vi "Device Settings Window.vi"(8 "Error In":errorcluster) -> (0 "Error Out":errorcluster)   [LabVIEW 2019]
uses:
  Controls/Device Settings.ctl
panel:
  in  "Device Settings":T1={"Device Type"="", "Device Name"="", "DAQmx Name"="Dev1", "Terminal Wiring"=10106} {"Terminal Wiring" items=["Default"=-1, "RSE"=10083, "NRSE"=10078, "Differential"=10106, "Pseudodifferential"=12529]}
  in  "Cancel Button":bool
  in  "OK Button":bool
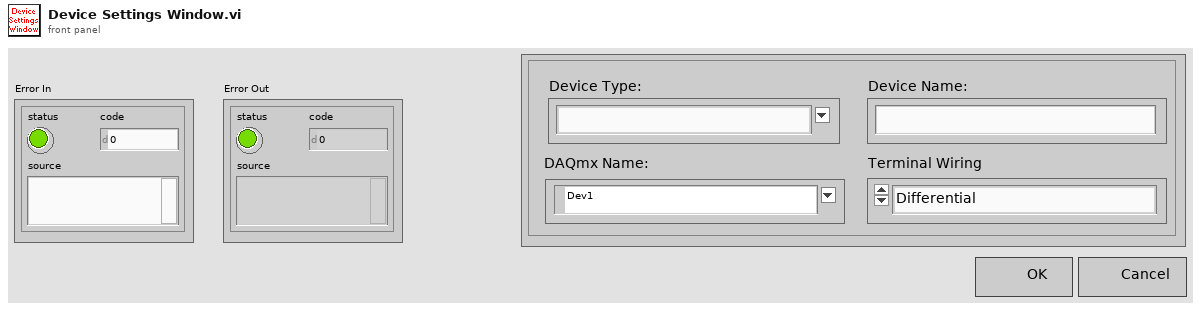
[diagram p1: front panel]
types:
  T1 = typedef "Device Settings.ctl" = cluster{"Device Type":string, "Device Name":string, "DAQmx Name":tag, "Terminal Wiring":i32}
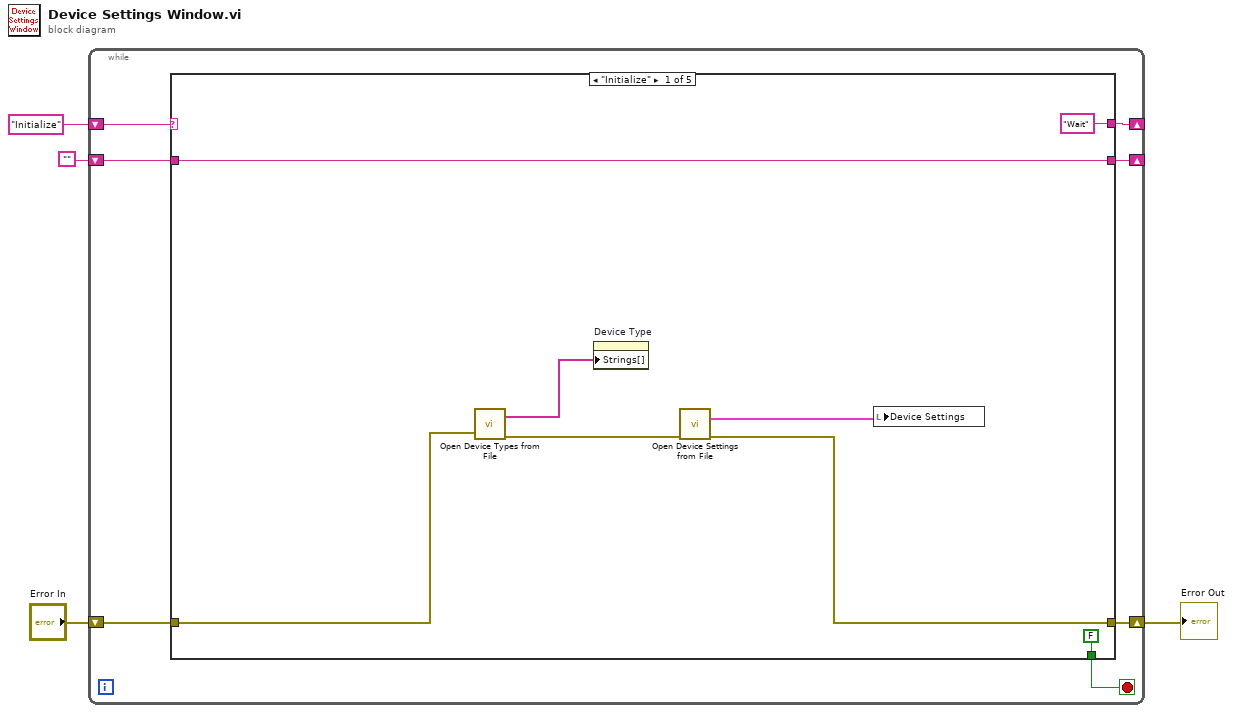
[diagram p0: block diagram]
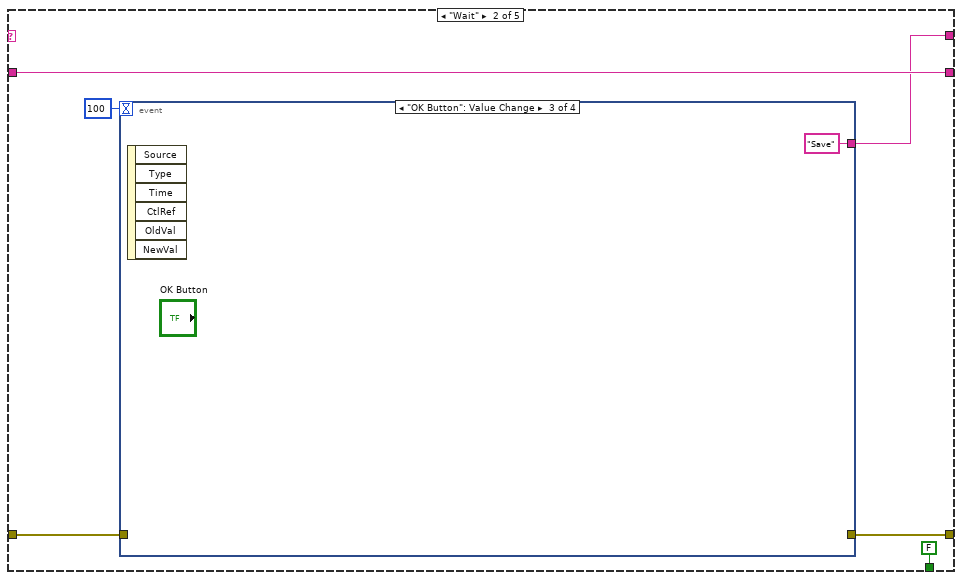
[diagram p2: hidden frame]
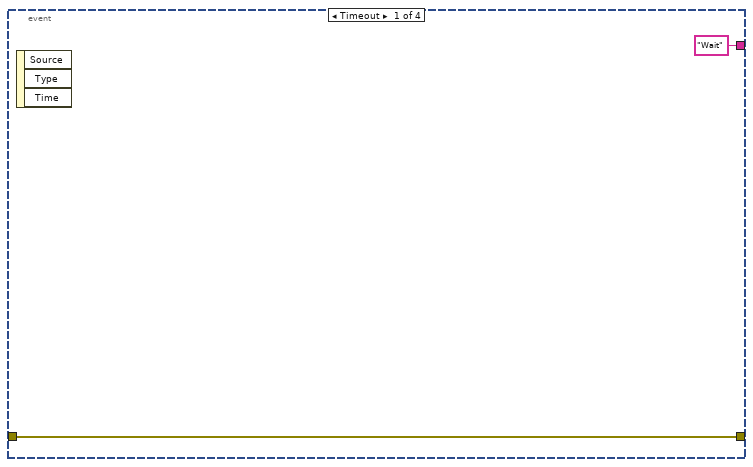
[diagram p3: hidden frame]
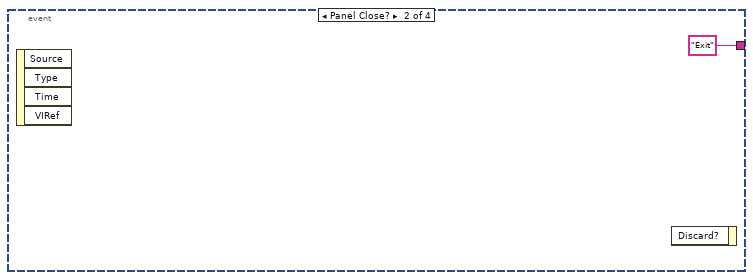
[diagram p4: hidden frame]
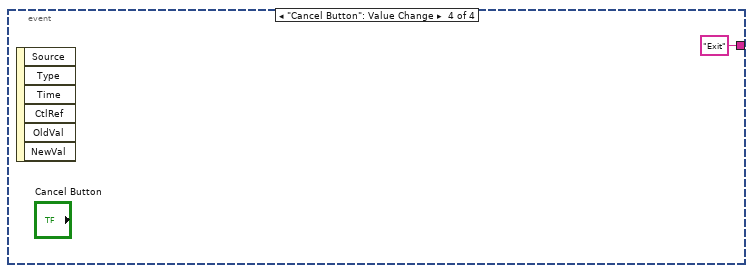
[diagram p5: hidden frame]
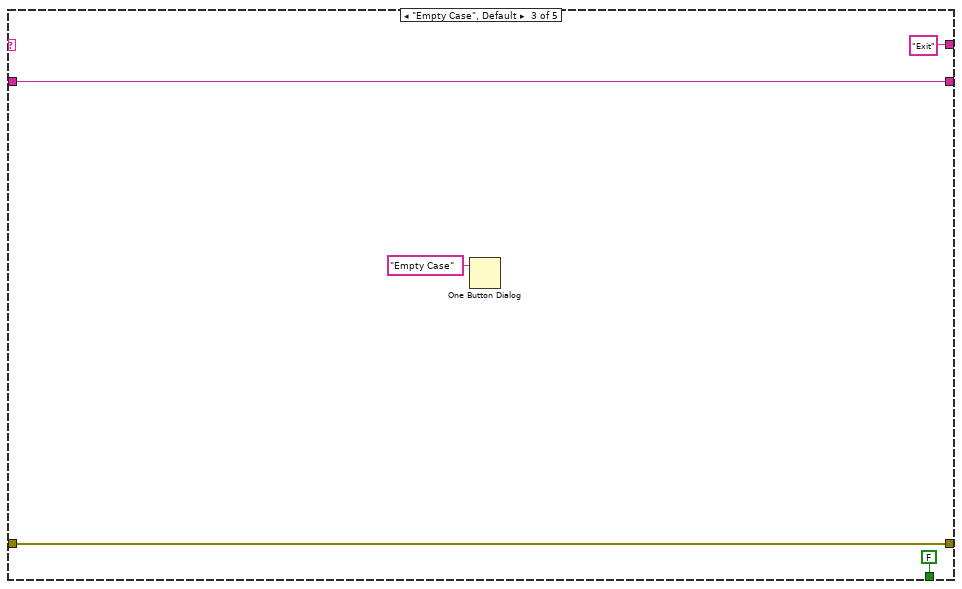
[diagram p6: hidden frame]
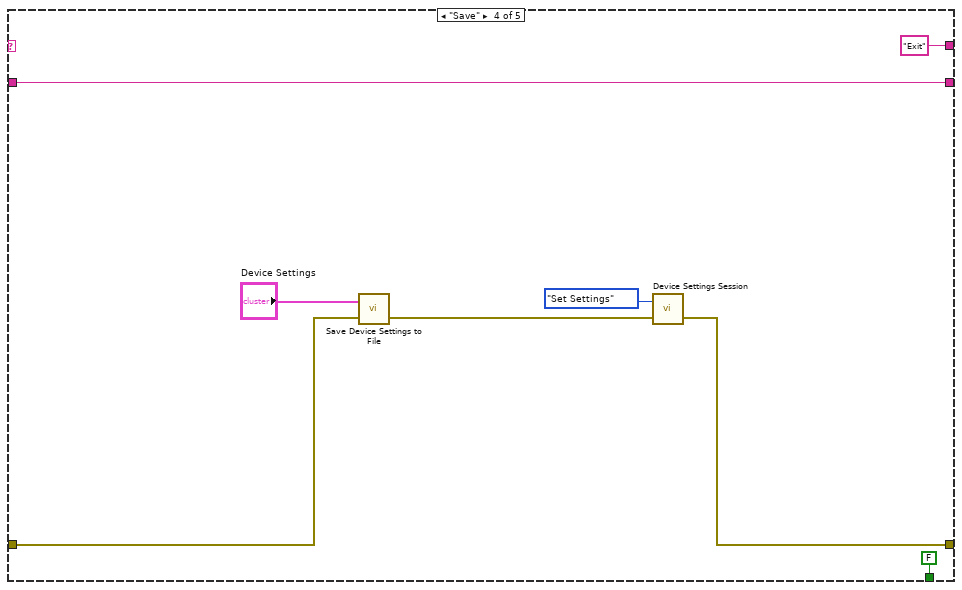
[diagram p7: hidden frame]
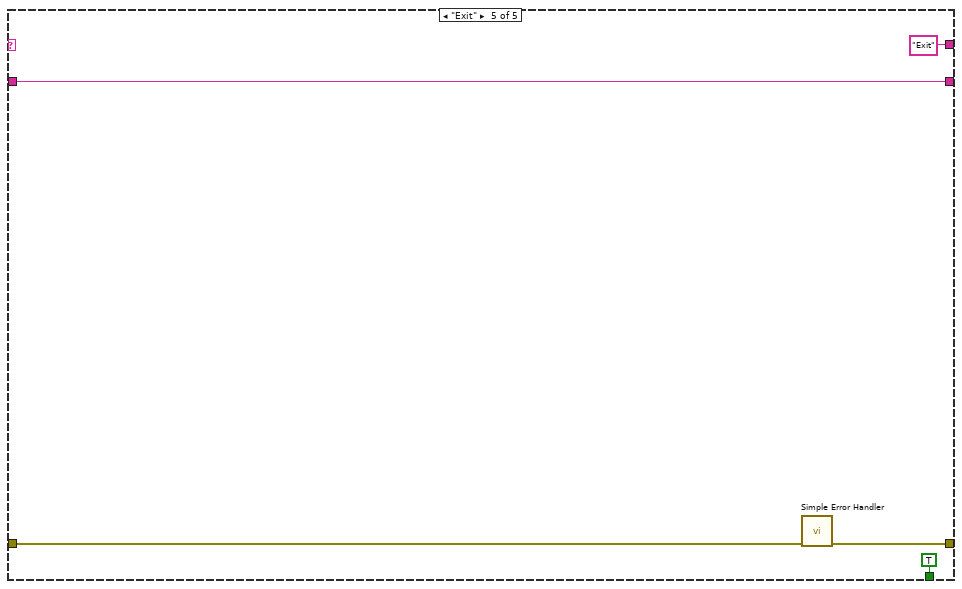
[diagram p8: hidden frame]
diagram:
  n1 = while {
    shift-right: [w7] -> _
    shift-left: "Initialize" ("key") -> [w11]
    shift-right: [w8] -> _
    shift-left: "" -> [w10]
    shift-right: [w5] -> w2
    shift-left: "Error In" -> [w9]
    stop <- w6 stop-if-true
    n2 = case shown="\"Initialize\"" w11 {
      tunnel: w10 -> [w17 w24 w32 w41 w48]
      tunnel: w9 -> [w16 w21 w33 w37 w45]
      tunnel: [w17 w24 w32 w41 w48] -> w8
      tunnel: ["Wait" ("key") w23 "Exit" ("key") "Exit" ("key") "Exit" ("key")] -> w7
      tunnel: [FALSE FALSE FALSE FALSE TRUE] -> w6
      tunnel: [w13 w20 w33 w36 w44] -> w5
      frame "Initialize" {
        n3 = call "Open Device Types from File.vi"("Error In"=w16) -> ("Error Out"=w14:errorcluster, "Device Types"=w15:string[])  [unwired: 1 in]
        n4 = property on="Device Type" class="CmbBox"("Strings[]"=w15) -> ()  [unwired: 2 in, 2 out]
        n5 = call "Open Device Settings from File.vi"("Error In"=w14) -> ("Device Settings"=w12:T1, "Error Out"=w13:errorcluster)  [unwired: 13 in]
        n6 = local write "Device Settings"(w12) -> ()
      }
      frame "Wait" {
        n7 = event shown="[2] \"OK Button\": Value Change" {
          selector: _ -> [_ _ _ _]
          dyn-events: _ -> [_ _ _ _]
          timeout: 100 -> [_ _ _ _]
          tunnel: ["Wait" ("key") "Exit" ("key") "Save" ("key") "Exit" ("key")] -> w23
          tunnel: w21 -> [w26 _ _ _]
          tunnel: [w26 _ _ _] -> w20
          event Timeout {
            n8 = event-data() -> ()  [unwired: 1 in, 3 out]
          }
          event Panel Close? {
            n9 = event-data() -> ()  [unwired: 1 in, 4 out]
            n10 = event-data() -> ()  [unwired: 2 in, 1 out]
          }
          event "OK Button": Value Change {
            n11 = event-data() -> ()  [unwired: 1 in, 6 out]
          }
          event "Cancel Button": Value Change {
            n12 = event-data() -> ()  [unwired: 1 in, 6 out]
          }
        }
      }
      frame "Empty Case", Default {
        n13 = One Button Dialog(message="Empty Case") -> ()  [unwired: 1 in, 1 out]
      }
      frame "Save" {
        n14 = call "Save Device Settings to File.vi"("Error In"=w37, "Device Settings"="Device Settings") -> ("Error Out"=w38:errorcluster)  [unwired: 1 in]
        n15 = call "Device Settings Session.vi"("Error In"=w38, "Type"=enum16{"Set Settings", "Get Settings"}."Set Settings") -> ("Error Out"=w36:errorcluster)  [unwired: 1 out]
      }
      frame "Exit" {
        n16 = call <vilib>:"Simple Error Handler.vi"("error in (no error)"=w45) -> ("error out"=w44:errorcluster)  [unwired: 4 in, 4 out]
      }
    }
  }
  "Error Out" <- w2
